vi "PS3 Controller.vi"(8 "error in (no error)":errorcluster) -> (0 "error out":errorcluster, 1 "direction info":T2, 2 "button info":T3, 3 "axis info":T4)   [LabVIEW 2014]
uses:
  <vilib>/Utility/inputDevices.llb/joystickAcquire.vi
  <vilib>/Utility/inputDevices.llb/closeJoystick.vi
panel:
  out "joystick info":T1(array[cluster])
  in  "stop":bool
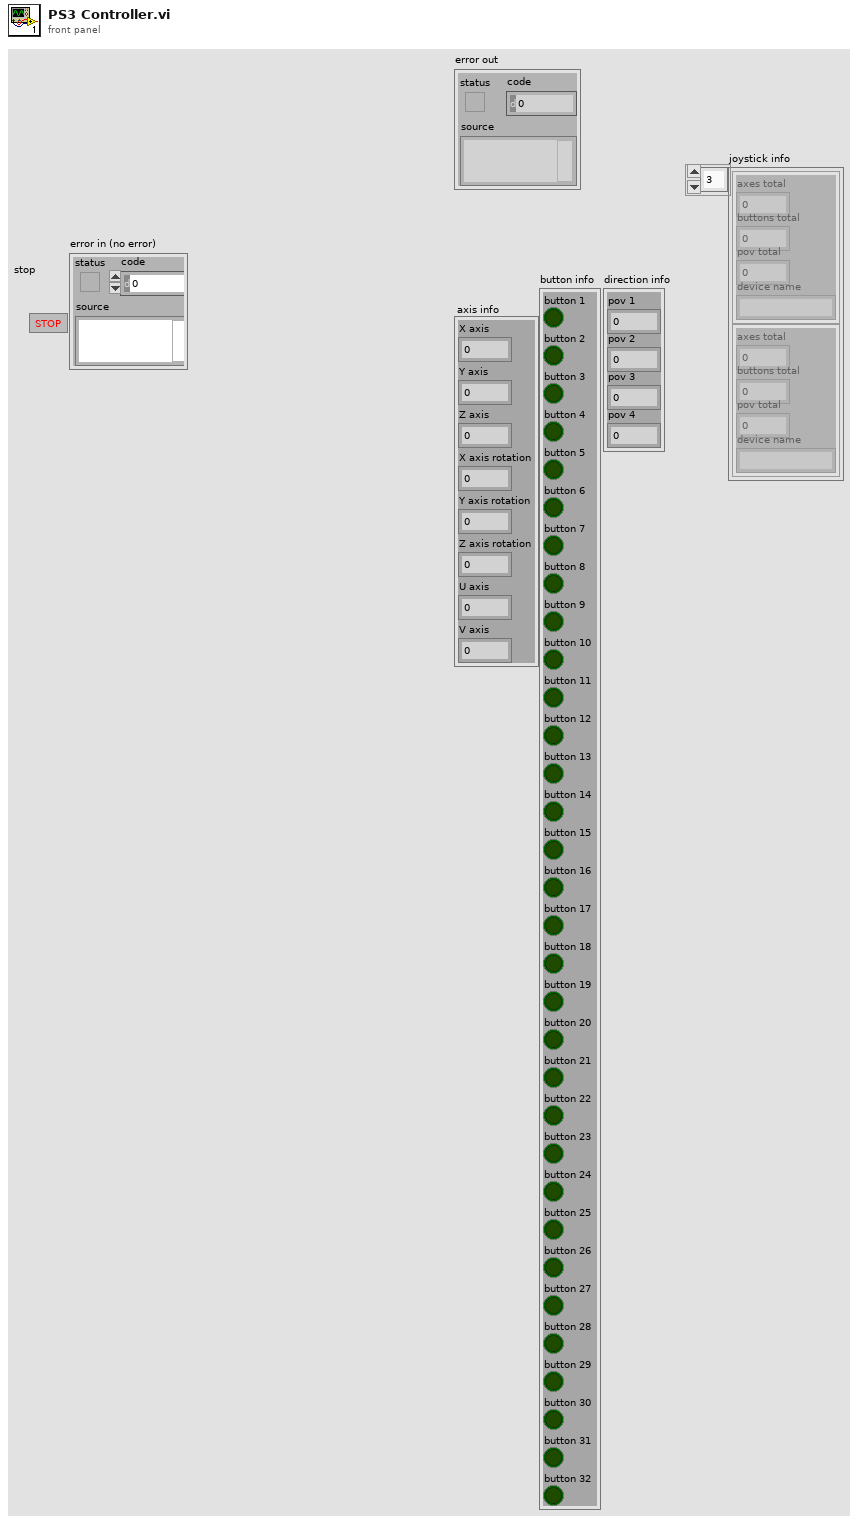
[diagram p1: front panel]
types:
  T1 = cluster{"axes total":u32, "buttons total":u32, "pov total":u32, "device name":string}[]
  T2 = cluster{"pov 1":i32, "pov 2":i32, "pov 3":i32, "pov 4":i32}
  T3 = cluster{"button 1":bool, "button 2":bool, "button 3":bool, "button 4":bool, "button 5":bool, "button 6":bool, "button 7":bool, "button 8":bool, "button 9":bool, "button 10":bool, "button 11":bool, "button 12":bool, "button 13":bool, "button 14":bool, "button 15":bool, "button 16":bool, "button 17":bool, "button 18":bool, "button 19":bool, "button 20":bool, "button 21":bool, "button 22":bool, "button 23":bool, "button 24":bool, "button 25":bool, "button 26":bool, "button 27":bool, "button 28":bool, "button 29":bool, "button 30":bool, "button 31":bool, "button 32":bool}
  T4 = cluster{"X axis":i32, "Y axis":i32, "Z axis":i32, "X axis rotation":i32, "Y axis rotation":i32, "Z axis rotation":i32, "U axis":i32, "V axis":i32}
  T5 = cluster{"X axis":dbl, "Y axis":dbl, "Z axis":dbl, "X axis rotation":dbl, "Y axis rotation":dbl, "Z axis rotation":dbl, "U axis":dbl, "V axis":dbl}
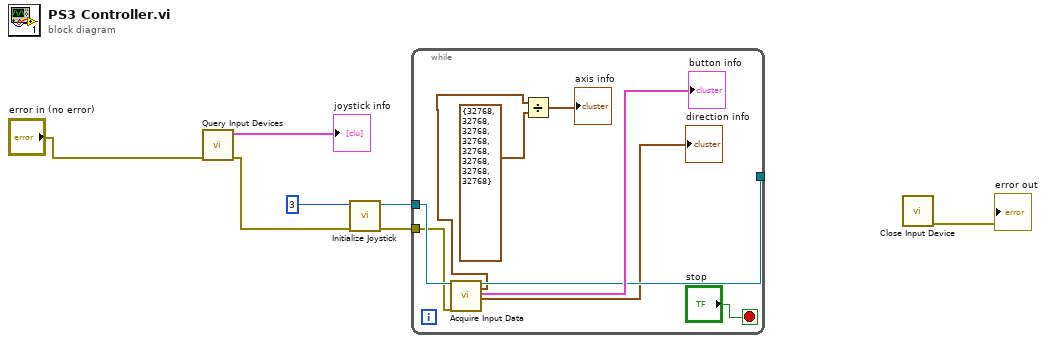
[diagram p0: block diagram]
diagram:
  n1 = call <vilib>:"Query Input Devices.vi"("error in (no error)"="error in (no error)") -> ("error out"=w2:errorcluster, "joystick info"=→"joystick info":T1)  [unwired: 7 in, 2 out]
  n2 = call <vilib>:"Initialize Joystick.vi"("error in (no error)"=w2, "device index"=3) -> ("error out"=w6:errorcluster, "device ID"=w7:refnum<k1>)  [unwired: 8 in]
  n3 = while {
    tunnel: w7 -> [w16]
    tunnel: w6 -> [w11]
    tunnel: [w14] -> _
    stop <- "stop" stop-if-true
    n4 = call-poly <vilib>:"Acquire Input Data.vi"("device ID"=w16, "error in (no error)"=w11) -> ("device ID"=w14:refnum<k1>, "axis info"=w9:T4, "button info"=→"button info":T3, "direction info"=→"direction info":T2)  [unwired: 13 in, 1 out]
    n5 = Divide(x=w9, y=T4 {"X axis"=32768, "Y axis"=32768, "Z axis"=32768, "X axis rotation"=32768, "Y axis rotation"=32768, "Z axis rotation"=32768, "U axis"=32768, "V axis"=32768}) -> (x/y=→"axis info":T5)
  }
  n6 = call-poly <vilib>:"Close Input Device.vi"() -> ("error out"=→"error out":errorcluster)  [unwired: 10 in]
